vi "Destroy User Events.vi"(8 "error in (no error)":errorcluster, 11 "Image Acquisition in":refnum<class "Image Acquisition.lvclass">) -> (0 "error out":errorcluster, 3 "Image Acquisition out":refnum<class "Image Acquisition.lvclass">)   [LabVIEW 2019, in "Image Acquisition.lvlib" / "Image Acquisition.lvclass"]
uses:
  Image Acquisition.lvclass
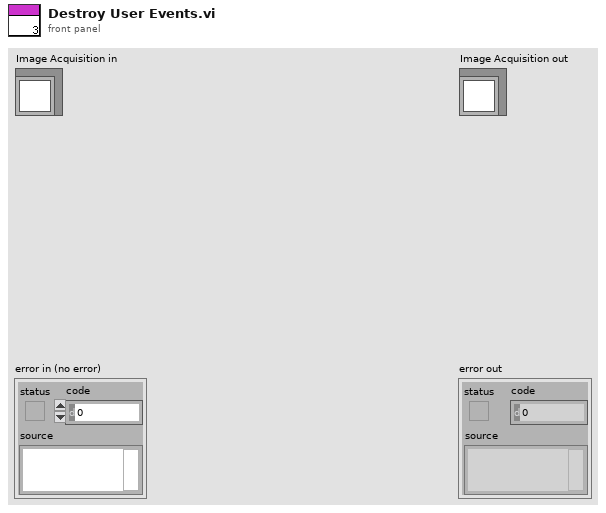
[diagram p1: front panel]
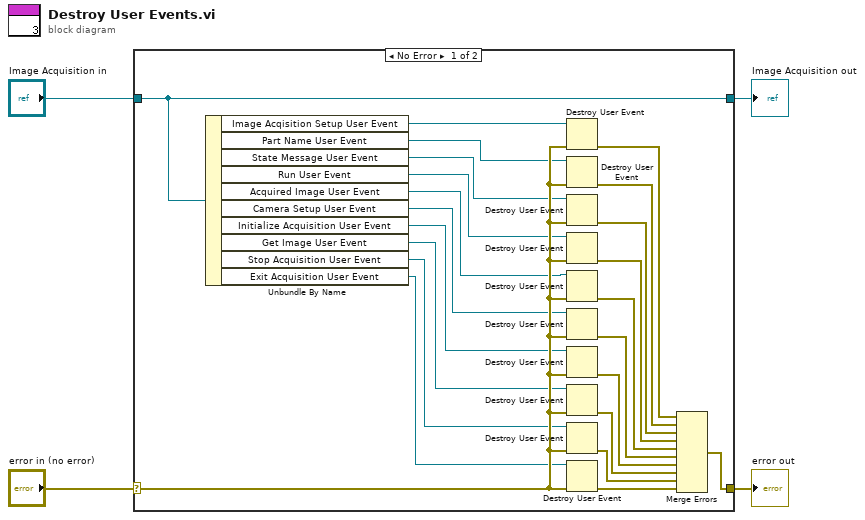
[diagram p0: block diagram]
diagram:
  n1 = case shown="No Error" "error in (no error)" {
    selector: "error in (no error)" -> [w26 w29]
    tunnel: [w15 w29] -> w3
    tunnel: [w27 w28] -> w1
    tunnel: "Image Acquisition in" -> [w27 w28]
    frame No Error {
      n2 = Unbundle By Name(w27) -> ("Image Acqisition Setup User Event"=w5:refnum<user-event>, "Part Name User Event"=w6:refnum<user-event>, "State Message User Event"=w7:refnum<user-event>, "Run User Event"=w8:refnum<user-event>, "Acquired Image User Event"=w9:refnum<user-event>, "Camera Setup User Event"=w10:refnum<user-event>, "Initialize Acquisition User Event"=w11:refnum<user-event>, "Get Image User Event"=w12:refnum<user-event>, "Stop Acquisition User Event"=w13:refnum<user-event>, "Exit Acquisition User Event"=w14:refnum<user-event>)
      n3 = Destroy User Event(user event=w5, error in=w26) -> (error out=w16:errorcluster)
      n4 = Destroy User Event(user event=w6, error in=w26) -> (error out=w17:errorcluster)
      n5 = Destroy User Event(user event=w7, error in=w26) -> (error out=w18:errorcluster)
      n6 = Destroy User Event(user event=w8, error in=w26) -> (error out=w19:errorcluster)
      n7 = Destroy User Event(user event=w9, error in=w26) -> (error out=w20:errorcluster)
      n8 = Destroy User Event(user event=w10, error in=w26) -> (error out=w21:errorcluster)
      n9 = Destroy User Event(user event=w11, error in=w26) -> (error out=w22:errorcluster)
      n10 = Destroy User Event(user event=w12, error in=w26) -> (error out=w23:errorcluster)
      n11 = Destroy User Event(user event=w13, error in=w26) -> (error out=w24:errorcluster)
      n12 = Destroy User Event(user event=w14, error in=w26) -> (error out=w25:errorcluster)
      n13 = Merge Errors(w16, w17, w18, w19, w20, w21, w22, w23, w24, w25) -> (w15:errorcluster)
    }
    frame Error {
    }
  }
  "error out" <- w3
  "Image Acquisition out" <- w1
